vi "接收参数处理.vi"(2 "输入参数数组":string[][](array[string])=[["a", "b", "c", "d", "e"], ["1", "2", "3", "4", "5"]], 3 "参数字符串":string) -> (0 "输出参数数组":string[][](array[string])=[["a", "b", "c", "d", "e"], ["1", "2", "3", "4", "5"]], 1 "未知的参数":string)   [LabVIEW 2017]
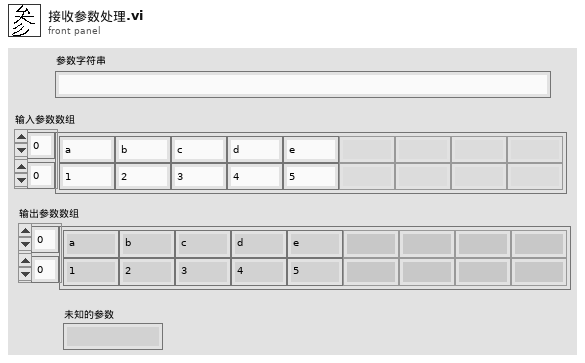
[diagram p1: front panel]
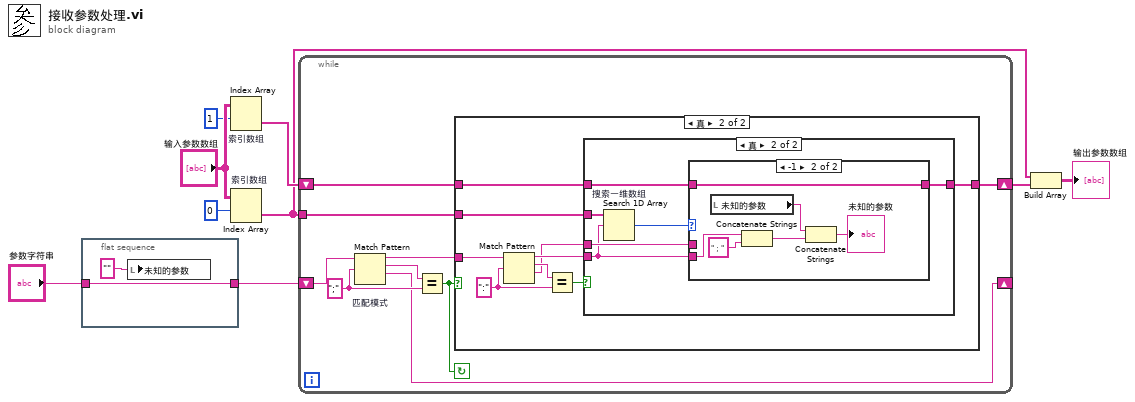
[diagram p0: block diagram]
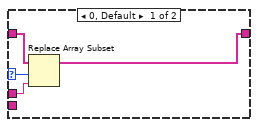
[diagram p4: hidden frame]
diagram:
  n1 = flat-sequence {
    tunnel: [w11] -> w9
    tunnel: "参数字符串" -> [w11]
    frame #0 {
      n2 = local write "未知的参数"("" ("未知的参数")) -> ()
    }
  }
  n3 = Index Array "索引数组"(array="输入参数数组", index (row)=1 ("索引 (行)")) -> (element=w5:string[])  [unwired: 1 in]
  n4 = Index Array "索引数组"(array="输入参数数组", index (row)=0 ("索引 (行)")) -> (element=w3:string[])  [unwired: 1 in]
  n5 = while {
    shift-right: [w16] -> _
    shift-left: w9 -> [w20]
    tunnel: w3 -> [w14]
    shift-right: [w13] -> w2
    shift-left: w5 -> [w15]
    stop <- w12 continue-if-true
    w18 = ";" ("正则表达式")
    n6 = Match Pattern "匹配模式"(string=w20, regular expression=w18) -> (before substring=w17:string, match substring=w19:string, after substring=w16:string)  [unwired: 1 in, 1 out]
    n7 = Equal?(x=w19, y=w18) -> (x = y?=w12:bool)
    n8 = case shown="真" w12 {
      tunnel: w17 -> [_ w30]
      tunnel: w15 -> [w21 w24]
      tunnel: w14 -> [_ w23]
      tunnel: [w21 w22] -> w13
      frame False {
      }
      frame True {
        w28 = ":" ("正则表达式")
        n9 = Match Pattern(string=w30, regular expression=w28) -> (before substring=w27:string, match substring=w29:string, after substring=w26:string)  [unwired: 1 in, 1 out]
        n10 = Equal?(x=w29, y=w28) -> (x = y?=w25:bool)
        n11 = case shown="真" w25 {
          tunnel: w27 -> [_ w32]
          tunnel: w26 -> [_ w36]
          tunnel: w23 -> [_ w35]
          tunnel: w24 -> [w31 w34]
          tunnel: [w31 w33] -> w22
          frame False {
          }
          frame True {
            n12 = Search 1D Array "搜索一维数组"(1D array=w35, element=w32) -> (index of element=w37:i32)  [unwired: 1 in]
            n13 = case shown="-1" w37 {
              selector: w37 -> [w40 _]
              tunnel: w34 -> [w41 w47]
              tunnel: w36 -> [w39 _]
              tunnel: [w38 w47] -> w33
              tunnel: w32 -> [_ w43]
              frame 0, Default {
                n14 = Replace Array Subset(array=w41, new element=w39, index=w40) -> (w38:string[])
              }
              frame -1 {
                n15 = local read "未知的参数"() -> (w46:string)
                n16 = Concatenate Strings(w43, "；" ("字符串")) -> (w44:string)
                n17 = Concatenate Strings(w46, w44) -> (→"未知的参数":string)
              }
            }
          }
        }
      }
    }
  }
  n18 = Build Array(w3, w2) -> (→"输出参数数组":string[][])
